vi "Change in Custom Action Definition.vi"(8 "error in (no error)":errorcluster, 9 "Custom Action":T1, 10 "Selected Custom Action File Name":string, 11 "Bundle Builder in":refnum<class "Bundle Builder.lvclass">) -> (0 "error out":errorcluster, 3 "Bundle Builder out":refnum<class "Bundle Builder.lvclass">)   [LabVIEW 2020, in "Bundle Builder.lvclass"]
uses:
  Bundle Builder.lvclass
  Bundle Builder.lvclass/Bundle Builder.ctl
  52107b19-8a4d-43d0-8707-c8fd6ef986f9.vi
  <vilib>/Comparison/Equal/Equal Functor/Equal Functor.lvclass
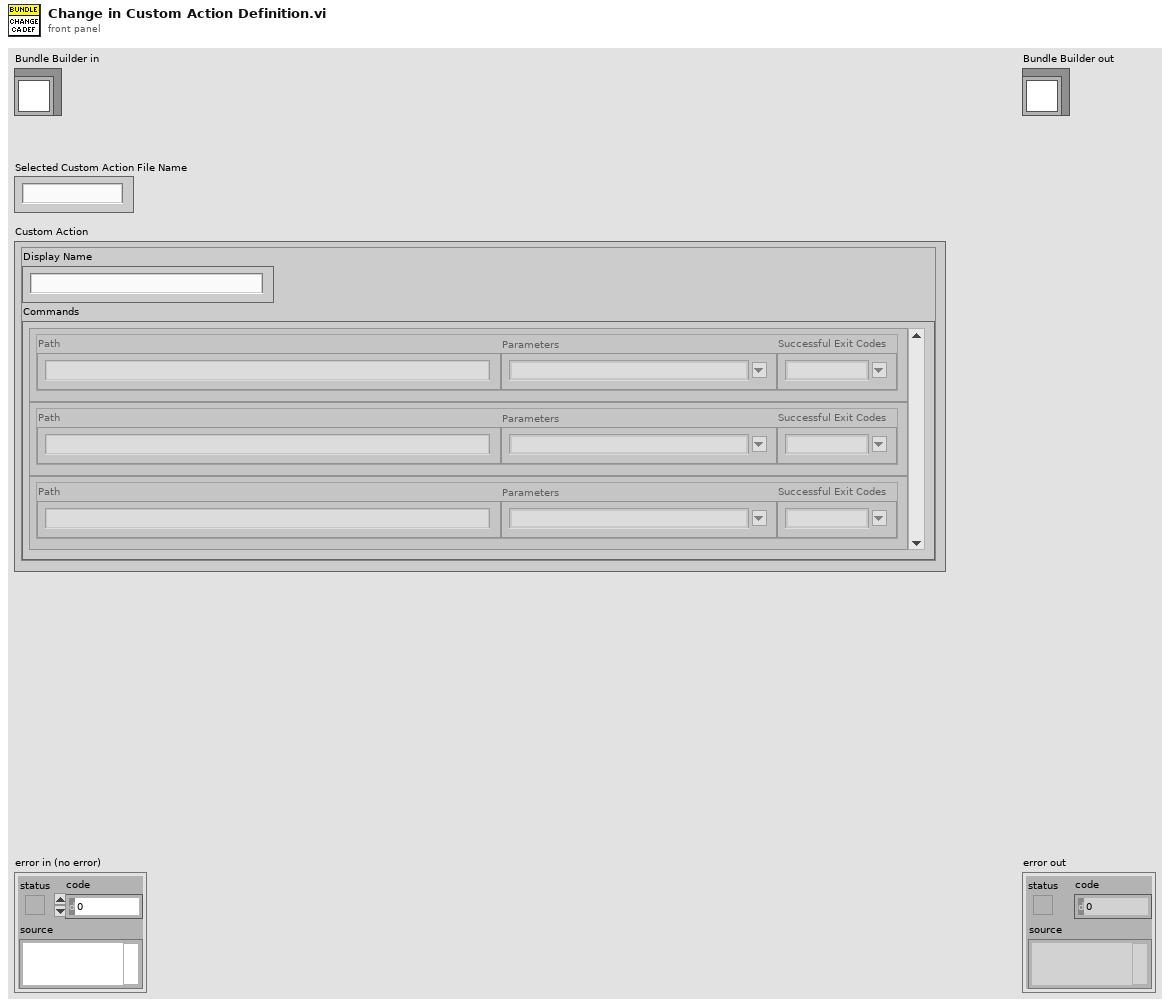
[diagram p1: front panel]
types:
  T1 = cluster{"Display Name":string, "Commands":cluster{"Path":string, "Parameters":string, "Successful Exit Codes":string}[]}
  T2 = cluster{"Display Name":string, "Commands":cluster{"Path":string, "Parameters":string, "Successful Exit Codes":string}[]}[]
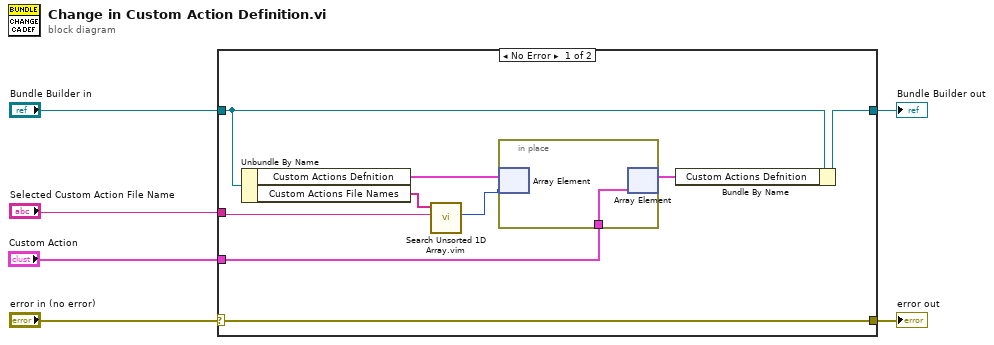
[diagram p0: block diagram]
diagram:
  n1 = case shown="No Error" "error in (no error)" {
    selector: "error in (no error)" -> [w15 w18]
    tunnel: [w15 w18] -> w5
    tunnel: [w14 w17] -> w3
    tunnel: "Bundle Builder in" -> [w13 w17]
    tunnel: "Selected Custom Action File Name" -> [w11 _]
    tunnel: "Custom Action" -> [w8 _]
    frame No Error {
      n2 = Unbundle By Name(w13) -> ("Custom Actions Defnition"=w10:T2, "Custom Actions File Names"=w12:string[])
      n3 = call "Search Unsorted 1D Array.vim"("element"=w11, "unsorted 1D array"=w12) -> ("index of element"=w9:i32)  [unwired: 9 in]
      n4 = in-place {
        in-place-border: w8 -> [w16]
        n5 = in-place-array #1(w10, w9) -> ()  [unwired: 1 out]
        n6 = in-place-array #1(w16) -> (w7:T2)  [unwired: 1 out]
      }
      n7 = Bundle By Name(cluster=w13, "Custom Actions Defnition"=w7) -> (w14:refnum<class "Bundle Builder.lvclass">)
    }
    frame Error {
    }
  }
  "error out" <- w5
  "Bundle Builder out" <- w3
